vi "Plate Tank 6.vi"() -> ()   [LabVIEW 2019]
uses:
  <vilib>/NI/Current Value Table/Type Defs/Single Tag.ctl
  <vilib>/NI/Current Value Table/Type Defs/Data Types.ctl
  <vilib>/NI/STM/TCP/Read Meta Data (TCP Ref).vi
  <vilib>/NI/STM/TCP/Get Connection Reference (TCP).vi
  <vilib>/NI/AMC/Read Termination Message.vi
  <vilib>/NI/AMC/Create Single Message.vi
  <vilib>/NI/AMC/Update Message Routing Info.vi
  <vilib>/NI/STM/TCP/Read Meta Data (TCP Clst).vi
  <vilib>/NI/AMC/Send Message.vi
  <vilib>/NI/AMC/Globals.vi
  <userlib>/_OpenG.lib/comparison/comparison.llb/I32 Changed__ogtk.vi
  <vilib>/NI/STM/TCP/Write Message (TCP).vi
  <vilib>/NI/AMC/AMC.lvlib
  <vilib>/NI/STM/NI STM.lvlib
  <vilib>/NI/Current Value Table/Current Value Table.lvlib
panel:
  out "Loaded Recipe":string
  in  "Override Motion":bool
  in  "Reverse Current Multiplier":dbl=3.0 min=0.1 max=100.0 step=0.01 format="%.2g"
  in  "Load A Recipe":bool
  in  "Save This Recipe":bool
  out "Right Time":dbl format="%.1f"
  out "Left Time":dbl format="%.1f"
  out "Total Amp*min R":dbl format="%.1f"
  out "Total Amp*min L":dbl format="%.1f"
  in  "Rectifer Settings":i32(listbox)
  in  "MO":string
  in  "BasT1_P Last Hr":bool
  in  "BasT1_Level Last Hr":bool
  out "Boolean 5":bool
  out "SumpBottom":bool
  out "Process 1 Supply":bool
  out "Sump Return":bool
  out "Boolean 2":bool
  out "SG":dbl format="%.3g"
  out "Return to sump 4":bool
  in  "Rectifer Data":enum32{"Standard", "Eng"}(tab)
  out "Current Step":i32
  out "Left Anode Actual Current":dbl(knob) scale=0.0..150.0
  out "Right Anode Actual Current":dbl(knob) scale=0.0..150.0
  out "Left Anode Amp-min":dbl(slide) scale=0.0..800.0
  out "Right Anode Amp-min":dbl(slide) scale=0.0..233.60000610351562
  out "Output Voltage":cluster{dbl, dbl}(graph)
  in  "Tab Control 2":enum32{"Standard", "ENG"}(tab)
  in  "Level Last Hr":bool
  out "Supply Flow":dbl(knob) scale=0.0..65.0
  out "Plating Cell Liquid Level":dbl(slide) scale=0.0..75.0
  out "Cell Temperature":dbl(slide) scale=0.0..60.0
  in  "Cell T Last Hr":bool
  out "Suck Pump":bool
  out "Suck Pump Flow":dbl format="%#_4g"
  out "SuckPipe":bool
  out "SuckPipe 3":bool
  out "Drain Tee Top":bool
  out "Return to sump 2":bool
  out "Return to sump 3":bool
  in  "Supply Tot FlwLast Hr":bool
  in  "Suck FlwLast Hr":bool
  out "Flow Controller":dbl(knob) scale=0.0..100.0
  in  "Tab Control":enum32{"Main Pump", "Suck Pump"}(tab)
  out "Amps":dbl format="%#.2g"
  out "Volts":dbl format="%#.1f"
  out "VFD T":dbl format="%#.2g"
  out "RPM":dbl format="%#.0f"
  out "Fault Code":dbl format="%#.2g"
  out "Freq":dbl format="%#.2g"
  out "SP1 Amps":dbl caption="Amps" format="%#.2g"
  out "SP1 Volts":dbl caption="Volts" format="%#.1g"
  out "SP1 RPM":dbl caption="RPM" format="%#.2g"
  out "SP1 VFD T":dbl caption="VFD T" format="%#.2g"
  out "SP1 Fault Code":dbl caption="Fault Code" format="%#.2g"
  out "SP1 Freq":dbl caption="Freq" format="%#.2g"
  out "Flow 1":dbl format="%#_4g"
  out "Flow 2":dbl format="%#_4g"
  out "Flow 3":dbl format="%#_4g"
  out "Flow 4":dbl format="%#_4g"
  out "Return to sump":bool
  out "E Stop":bool
  out "Run Enabled?":bool
  in  "Full Drain Plating Cell":bool
  out "Rack Motion":bool
  out "Right Eductor Motion":bool
  out "Left Eductor Motion":bool
  out "Right Output On":bool
  in  "Enable Rack Motion":bool
  in  "Rack RPM":dbl(knob) scale=0.0..15.0
  out "Left Output On":bool
  in  "Start Cycle":bool
  in  "Cancel Cycle":bool
  out "SuckPipe 2":bool
  out "Main Pump":bool
  in  "Enable Eductor Motion":bool
  in  "Eductor RPM":dbl(knob) scale=0.0..15.0
  in  "Supply Pressure (kPa)":dbl(knob)=50.0 min=50.0 max=200.0 step=5.0 scale=50.0..200.0
  in  "Total Inflow (L/min)":dbl(knob)=40.0 min=25.0 max=50.0 step=0.5 scale=25.0..50.0
  in  "Suck Pump fraction of inflow":dbl(knob)=5.0 min=5.0 max=90.0 step=1.0 scale=0.0..90.0
  out "Sump Level":dbl(slide) scale=0.0..1000.0
  out "Supply Pressure":dbl(knob) scale=0.0..200.0
  in  "Enable Suck Pump":bool
  in  "Enable Plating Cell":bool
  in  "Machine":bool
  in  "Basement 4":bool
  in  "Dryer":bool
  in  "Rinse 4":bool
  in  "Rinse 3":bool
  in  "Rinse 2":bool
  in  "Basement 3":bool
  in  "Basement 2":bool
  in  "Basement 1":bool
  in  "Plater 6":bool
  in  "Plater 5":bool
  in  "Plater 4":bool
  in  "Plater 3":bool
  in  "Plater 2":bool
  in  "Plater 1":bool
  in  "Predip":bool
  in  "Rinse 1":bool
  in  "Cleaner":bool
  in  "Etch":bool
  out "status":string
  out "Boolean 4":bool
  # "Module Selection"
  # "Rectifier Settings"
  # "Fluid Flow Control"
  # "Rectifier Control"
  # "Rectifier Output"
  # "Note: RPM settings shared with tank 6"
  # "Motion starts when rectifiers cycle"
  # "kPa"
  # "@"
  # "Output"
  # "cm"
  # "°C"
  # "L/min"
  # "cm"
  # "L/min"
  # "L/min"
  # "L/min"
  # "L/min"
  # "L/min"
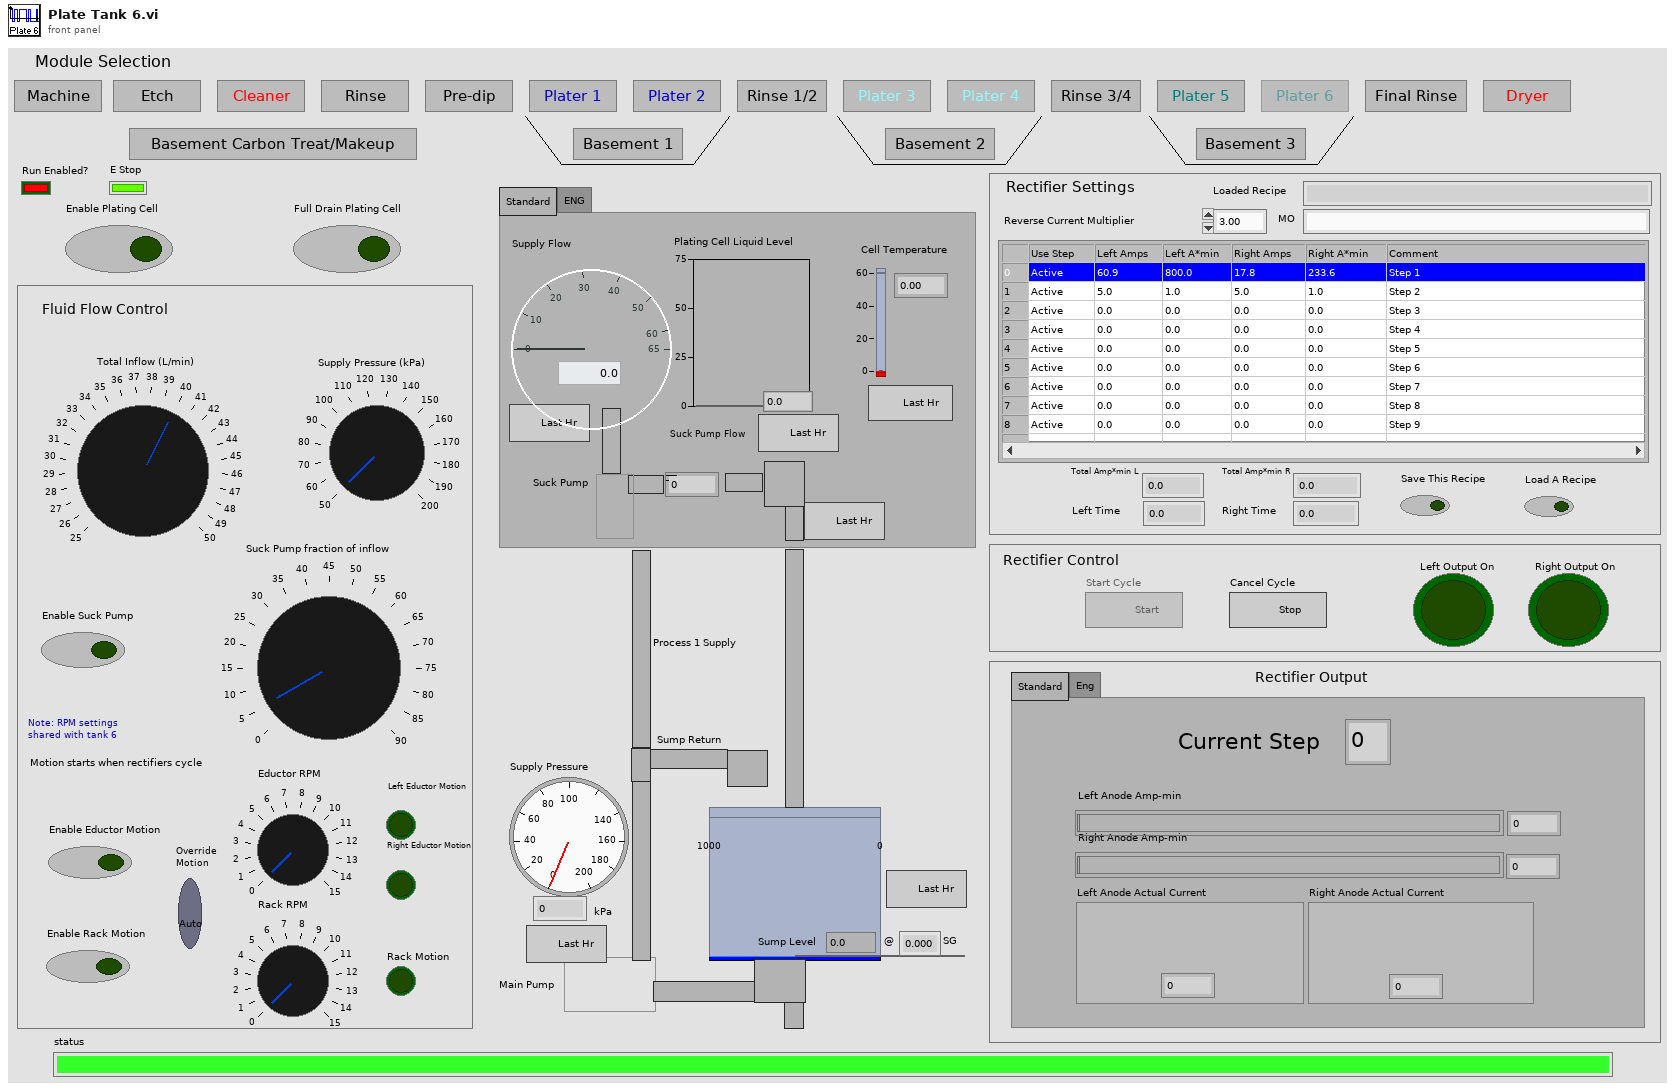
[diagram p1: front panel]
types:
  T1 = typedef "Current Value Table.lvlib/Single Tag.ctl" = cluster{"Data Type":T2, "Name":string, "Value":string, "Description":string}
  T2 = typedef "Current Value Table.lvlib/Data Types.ctl" = enum16{"Double", "Single", "I64", "I32", "I16", "I8", "U64", "U32", "U16", "U8", "String", "Boolean", "Array of U8", "Array of U16", "Array of U32", "Array of U64", "Array of I64", "Array of I32", "Array of I16", "Array of I8", "Array of Double", "Array of Single", "Array of Boolean", "Array of String"}
  T3 = typedef "NI STM.lvlib/TCP Connection Info.ctl" = cluster{"connection ID":refnum<k5>, "meta data":T4[]}
  T4 = typedef "NI STM.lvlib/MetaDataElement.ctl" = string
  T5 = typedef "AMC.lvlib/Message Queue.ctl" = refnum<queue>
  T6 = cluster{"Shift":bool, "Ctrl":bool, "Alt":bool, "Cmd":bool, "Opt":bool}
  T7 = typedef "LVPoint32TypeDef.ctl" = cluster{"Horizontal":i32, "Vertical":i32}
  T8 = typedef "LVRowAndColumnTypeDef.ctl" = cluster{"Row":i32, "Column":i32}
  T9 = enum8{"Enabled", "Disabled", "Disabled and Grayed Out"}
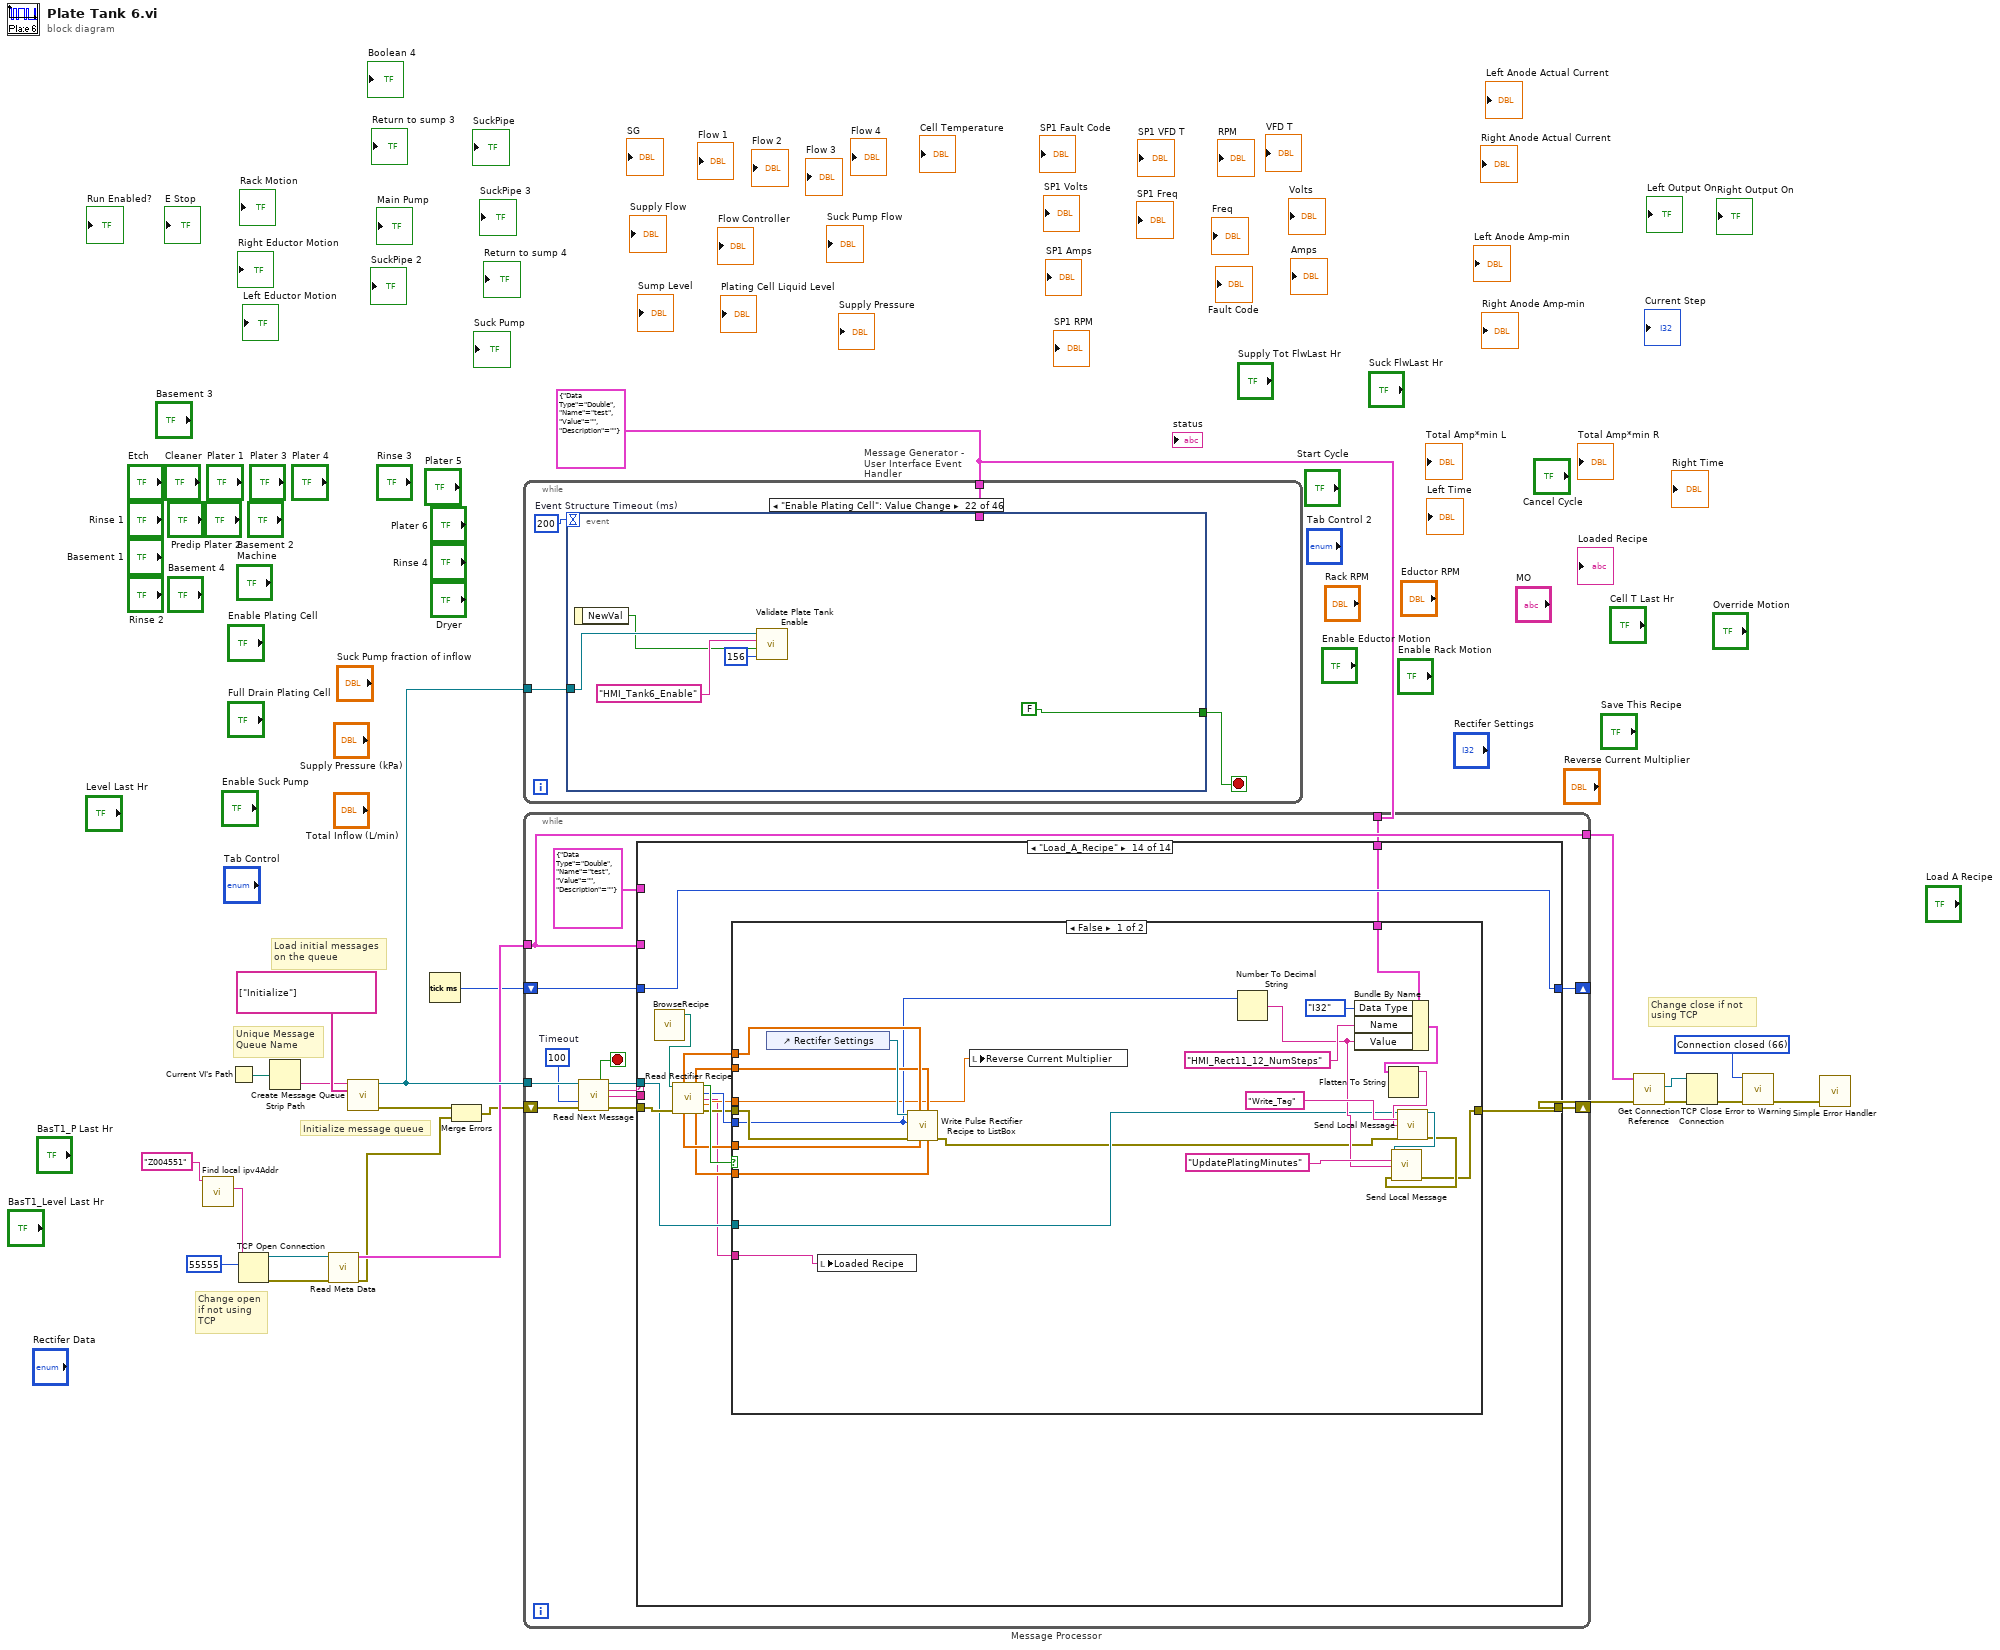
[diagram p0: block diagram]
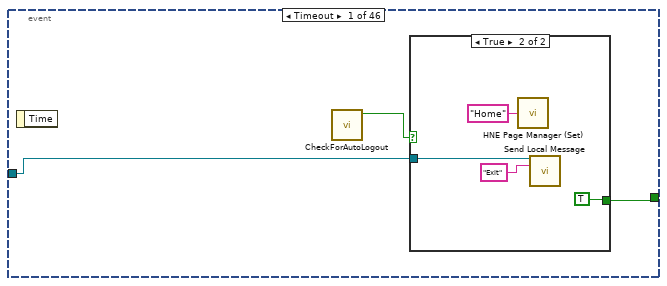
[diagram p2: hidden frame]
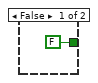
[diagram p3: hidden frame]
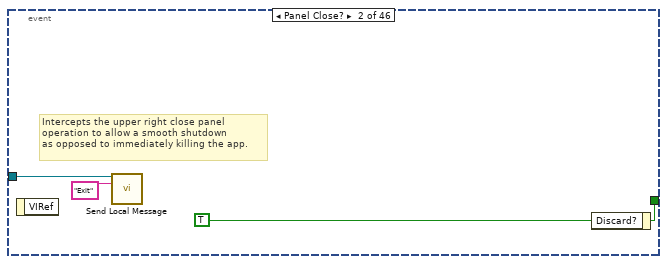
[diagram p4: hidden frame]
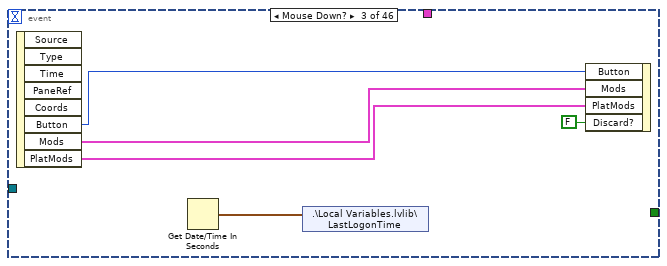
[diagram p5: hidden frame]
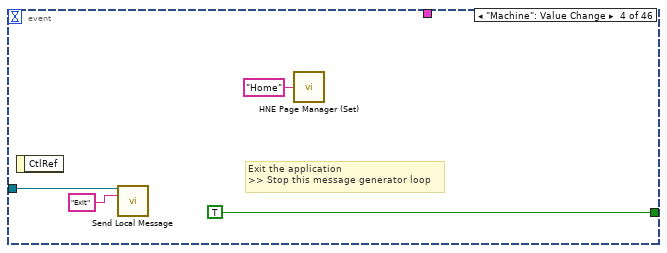
[diagram p6: hidden frame]
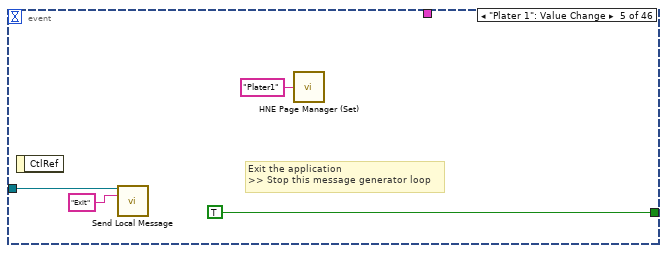
[diagram p7: hidden frame]
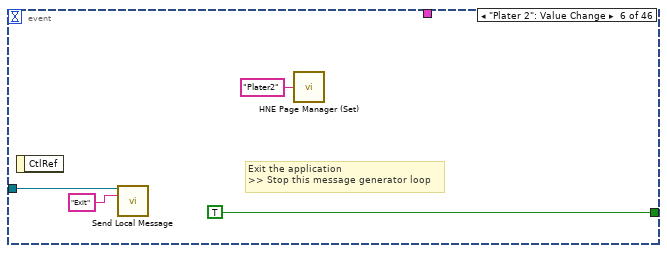
[diagram p8: hidden frame]
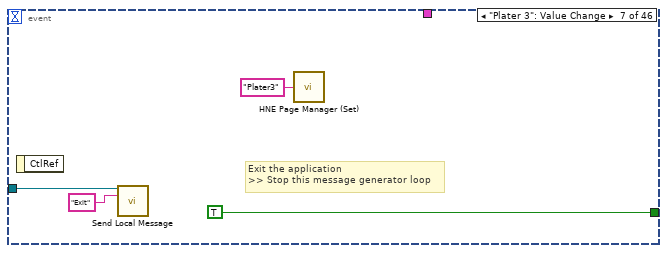
[diagram p9: hidden frame]
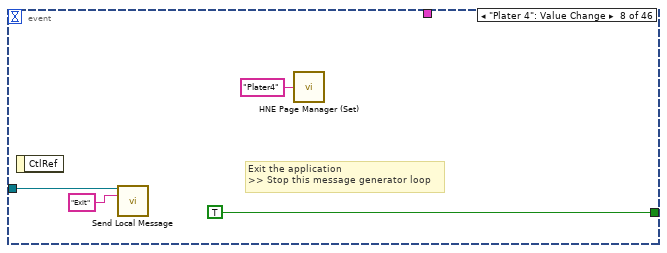
[diagram p10: hidden frame]
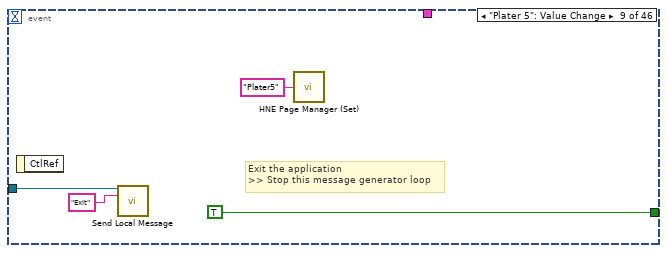
[diagram p11: hidden frame]
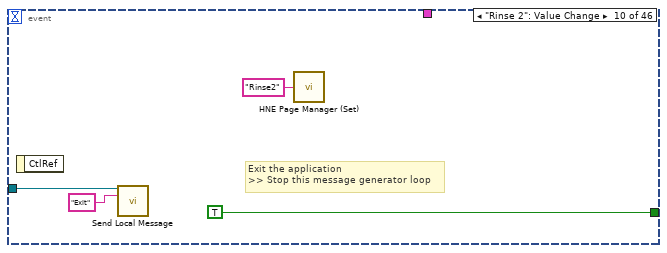
[diagram p12: hidden frame]
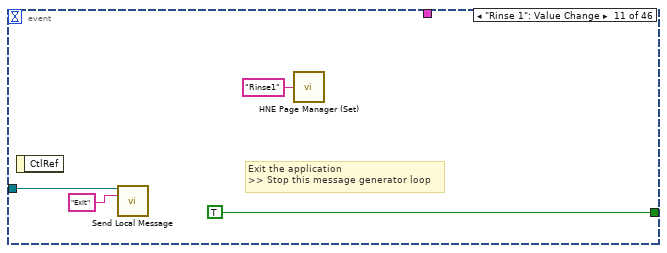
[diagram p13: hidden frame]
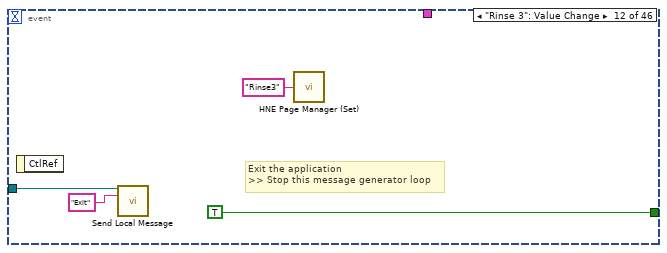
[diagram p14: hidden frame]
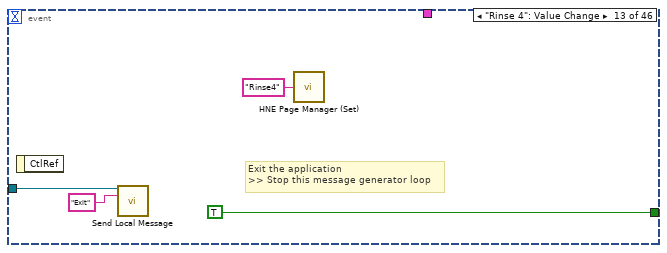
[diagram p15: hidden frame]
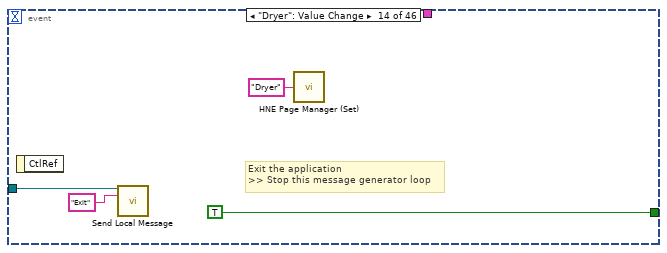
[diagram p16: hidden frame]
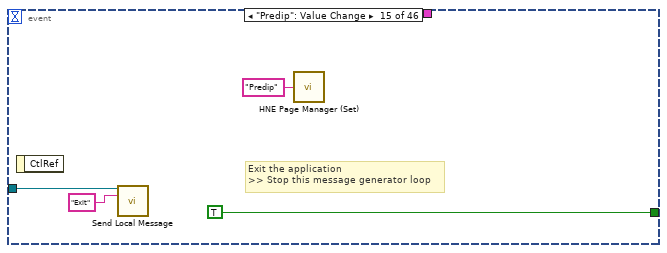
[diagram p17: hidden frame]
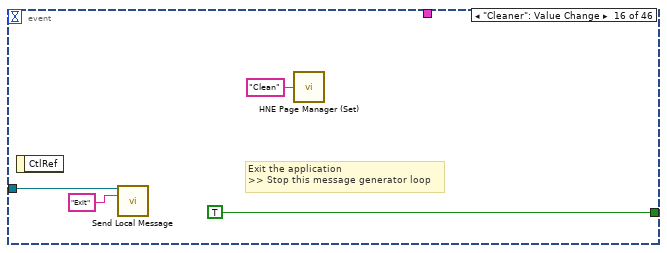
[diagram p18: hidden frame]
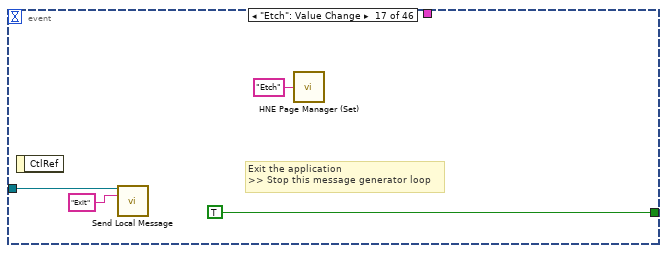
[diagram p19: hidden frame]
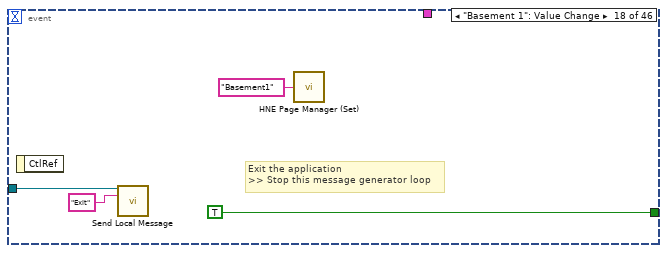
[diagram p20: hidden frame]
diagram:
  w1 = T1 {"Data Type"=enum."Double", "Name"="test", "Value"="", "Description"=""} ("Tag")
  w13 = 66 items=["No Error", "Argument Error", "Memory Full", "Out of Zone", "End of File", "File Already Open", "Generic File IO Error", "File Not Found", "File Permission Error", "Disk Full", "Duplicate Path", "Too Many Files Open", "Not Enabled", "Resource File Not Found", "Cannot Add Resource", "Resource Not Found", "Image Not Found", "Image Memory Error", "Pen Does Not Exist", "Config Bad Type", "Config Token Not Found", "Config Parse Error", "Config Memory Error", "Bad External Code Format", "Bad External Code Offset", "External Code Not Present", "Null Window", "Destroy Window Mixup", "Null Menu", "Print Aborted", "Bad Print Record", "Print Driver Error", "Windows Error During Print", "Memory Error During Print", "Print Dialog Error", "Generic Print Error", "Invalid Device Refnum", "Device Not Found", "Device Parameter Error", "Device Unit Error", "Can't Open Device", "Device Call Aborted", "Generic Error", "Cancelled By User", "Object ID Too Low", "Object ID Too High", "Object Not In Heap", "Unknown Heap", "Bad DefProc ID", "DefProc Not In Table", "Message Out Of Range", "Null Method", "Unknown Message", "Manager Call Not Supported", "Bad address", "Connection In progress", "Connection timed out", "Connection is already in progress", "Network attribute not supported", "Network error", "Address in use", "System out of memory", "Connection aborted", "Connection refused", "Connection is not connected", "Connection is already connected", "Connection closed", "Initialize error (interapplication manager)", "Bad occurrence", "Wait on unbound occurrence handler", "Occurrence queue overflow", "Bad path", "Semaphore not signaled", "Unrecognized type (interapplication manager)"] ("1st Error to Convert")
  # "Change close if not using TCP"
  # "Change open if not using TCP"
  # "Initialize message queue"
  # "Unique Message\nQueue Name"
  # "Load initial messages\non the queue"
  n1 = call "Find local ipv4Addr.vi"("MachineToFind"="Z004551" ("Target IP Address")) -> ("name"=w5:string)  [unwired: 9 in, 1 out]
  n2 = Current VI's Path() -> (path=w19:path)
  n3 = TCP Open Connection(address=w5, remote port or service name=u16 55555 ("remote port")) -> (connection ID=w17:refnum<k5>, error out=w16:errorcluster)  [unwired: 1 in, 2 out]
  n4 = Strip Path(path=w19) -> (name=w21:string)  [unwired: 1 out]
  n5 = call-poly <vilib>:"Read Meta Data.vi"("error in"=w16, "connection ID"=w17) -> ("error out"=w3:errorcluster, "connection info out"=w15:T3)  [unwired: 7 in, 1 out]
  n6 = call <vilib>:"Create Message Queue.vi"("message queue name"=w21, "initial message names"=string[] ["Initialize"]) -> ("message queue out"=w20:T5, "error out"=w4:errorcluster)  [unwired: 12 in]
  n7 = Tick Count (ms)() -> (millisecond timer value=w7:u32)
  n8 = Merge Errors(w4, w3) -> (w2:errorcluster)
  n9 = while "Message Generator - User Interface Event Handler" {
    tunnel: w20 -> [w24]
    tunnel: w1 -> [w23]
    stop <- w25 stop-if-true
    w26 = 200  # Event Structure Timeout (ms)
    n10 = event shown="[21] \"Enable Plating Cell\": Value Change" {
      selector: _ -> [_ _ _ _ _ _ _ _ _ _ _ _ _ _ _ _ _ _ _ _ _ _ _ _ _ _ _ _ _ _ _ _ _ _ _ _ _ _ _ _ _ _ _ _ _ _]
      dyn-events: _ -> [_ _ _ _ _ _ _ _ _ _ _ _ _ _ _ _ _ _ _ _ _ _ _ _ _ _ _ _ _ _ _ _ _ _ _ _ _ _ _ _ _ _ _ _ _ _]
      timeout: w26 -> [_ _ _ _ _ _ _ _ _ _ _ _ _ _ _ _ _ _ _ _ _ _ _ _ _ _ _ _ _ _ _ _ _ _ _ _ _ _ _ _ _ _ _ _ _ _]
      tunnel: [w29 w37 _ TRUE ("Discard?") TRUE ("Discard?") TRUE ("Discard?") TRUE ("Discard?") TRUE ("Discard?") TRUE ("Discard?") TRUE ("Discard?") TRUE ("Discard?") TRUE ("Discard?") TRUE ("Discard?") TRUE ("Discard?") TRUE ("Discard?") TRUE ("Discard?") TRUE ("Discard?") TRUE ("Discard?") TRUE ("Discard?") TRUE ("Discard?") TRUE ("Discard?") FALSE ("Discard?") FALSE ("Discard?") FALSE ("Discard?") FALSE ("Discard?") FALSE ("Discard?") FALSE ("Discard?") FALSE ("Discard?") FALSE ("Discard?") FALSE ("Discard?") FALSE ("Discard?") FALSE ("Discard?") FALSE ("Discard?") FALSE ("Discard?") FALSE ("Discard?") FALSE ("Discard?") _ _ _ _ _ _ _ _ _ _] -> w25
      tunnel: w24 -> [w28 w35 _ w44 w48 w52 w56 w60 w64 w68 w72 w76 w80 w84 w88 w92 w96 w100 w104 w108 w112 w118 w121 w126 w139 w150 w161 w172 w183 w187 w201 w221 w231 w241 w251 w263 w265 w267 w272 w277 w282 w287 w292 w299 w317 _]
      tunnel: w23 -> [_ _ _ _ _ _ _ _ _ _ _ _ _ _ _ _ _ _ _ _ _ _ _ _ w136 w147 w158 w169 w180 w186 w200 w220 w230 w240 w250 w262 _ _ _ _ _ _ _ w298 _ _]
      event Timeout {
        n11 = event-data() -> ()  [unwired: 2 out]
        n12 = call "CheckForAutoLogout.vi"() -> ("Boolean"=w27:bool)  [unwired: 11 in]
        n13 = case shown="True" w27 {
          tunnel: [FALSE ("Discard?") TRUE ("Discard?")] -> w29
          tunnel: w28 -> [_ w31]
          frame False {
          }
          frame True {
            n14 = call <userlib>:"HNE Page Manager (Set).vi"("Next Page"="Home") -> ()  [unwired: 4 in, 1 out]
            n15 = call <vilib>:"Send Local Message.vi"("message queue in"=w31, "message name"="Exit") -> ()  [unwired: 11 in, 3 out]
          }
        }
      }
      event Panel Close? {
        w37 = TRUE ("Discard?")
        # "Intercepts the upper right close panel\noperation to allow a smooth shutdown\nas opposed to immediately killing the app."
        n16 = event-data() -> ()  [unwired: 2 out]
        n17 = call <vilib>:"Send Local Message.vi"("message queue in"=w35, "message name"="Exit") -> ()  [unwired: 11 in, 3 out]
        n18 = event-data("Discard?"=w37) -> ()  [unwired: 1 in, 1 out]
      }
      event Mouse Down? {
        n19 = event-data() -> ("Button"=w41:u16, "Mods"=w40:cluster{"Double Click":bool, "Menu Key":bool}, "PlatMods"=w39:T6)  [unwired: 6 out]
        n20 = Get Date/Time In Seconds() -> (seconds since 1Jan1904=w38:timestamp)
        n21 = shared-variable ".\\Local Variables.lvlib\\LastLogonTime"(w38) -> ()  [unwired: 1 in, 1 out]
        n22 = event-data("Button"=w41, "Mods"=w40, "PlatMods"=w39, "Discard?"=FALSE) -> ()  [unwired: 1 in, 1 out]
      }
      event "Machine": Value Change {
        # "Exit the application\n>> Stop this message generator loop"
        n23 = event-data() -> ()  [unwired: 2 out]
        n24 = call <vilib>:"Send Local Message.vi"("message queue in"=w44, "message name"="Exit") -> ()  [unwired: 11 in, 3 out]
        n25 = call <userlib>:"HNE Page Manager (Set).vi"("Next Page"="Home") -> ()  [unwired: 4 in, 1 out]
      }
      event "Plater 1": Value Change {
        # "Exit the application\n>> Stop this message generator loop"
        n26 = event-data() -> ()  [unwired: 2 out]
        n27 = call <vilib>:"Send Local Message.vi"("message queue in"=w48, "message name"="Exit") -> ()  [unwired: 11 in, 3 out]
        n28 = call <userlib>:"HNE Page Manager (Set).vi"("Next Page"="Plater1") -> ()  [unwired: 4 in, 1 out]
      }
      event "Plater 2": Value Change {
        # "Exit the application\n>> Stop this message generator loop"
        n29 = event-data() -> ()  [unwired: 2 out]
        n30 = call <vilib>:"Send Local Message.vi"("message queue in"=w52, "message name"="Exit") -> ()  [unwired: 11 in, 3 out]
        n31 = call <userlib>:"HNE Page Manager (Set).vi"("Next Page"="Plater2") -> ()  [unwired: 4 in, 1 out]
      }
      event "Plater 3": Value Change {
        # "Exit the application\n>> Stop this message generator loop"
        n32 = event-data() -> ()  [unwired: 2 out]
        n33 = call <vilib>:"Send Local Message.vi"("message queue in"=w56, "message name"="Exit") -> ()  [unwired: 11 in, 3 out]
        n34 = call <userlib>:"HNE Page Manager (Set).vi"("Next Page"="Plater3") -> ()  [unwired: 4 in, 1 out]
      }
      event "Plater 4": Value Change {
        # "Exit the application\n>> Stop this message generator loop"
        n35 = event-data() -> ()  [unwired: 2 out]
        n36 = call <vilib>:"Send Local Message.vi"("message queue in"=w60, "message name"="Exit") -> ()  [unwired: 11 in, 3 out]
        n37 = call <userlib>:"HNE Page Manager (Set).vi"("Next Page"="Plater4") -> ()  [unwired: 4 in, 1 out]
      }
      event "Plater 5": Value Change {
        # "Exit the application\n>> Stop this message generator loop"
        n38 = event-data() -> ()  [unwired: 2 out]
        n39 = call <vilib>:"Send Local Message.vi"("message queue in"=w64, "message name"="Exit") -> ()  [unwired: 11 in, 3 out]
        n40 = call <userlib>:"HNE Page Manager (Set).vi"("Next Page"="Plater5") -> ()  [unwired: 4 in, 1 out]
      }
      event "Rinse 2": Value Change {
        # "Exit the application\n>> Stop this message generator loop"
        n41 = event-data() -> ()  [unwired: 2 out]
        n42 = call <vilib>:"Send Local Message.vi"("message queue in"=w68, "message name"="Exit") -> ()  [unwired: 11 in, 3 out]
        n43 = call <userlib>:"HNE Page Manager (Set).vi"("Next Page"="Rinse2") -> ()  [unwired: 4 in, 1 out]
      }
      event "Rinse 1": Value Change {
        # "Exit the application\n>> Stop this message generator loop"
        n44 = event-data() -> ()  [unwired: 2 out]
        n45 = call <vilib>:"Send Local Message.vi"("message queue in"=w72, "message name"="Exit") -> ()  [unwired: 11 in, 3 out]
        n46 = call <userlib>:"HNE Page Manager (Set).vi"("Next Page"="Rinse1") -> ()  [unwired: 4 in, 1 out]
      }
      event "Rinse 3": Value Change {
        # "Exit the application\n>> Stop this message generator loop"
        n47 = event-data() -> ()  [unwired: 2 out]
        n48 = call <vilib>:"Send Local Message.vi"("message queue in"=w76, "message name"="Exit") -> ()  [unwired: 11 in, 3 out]
        n49 = call <userlib>:"HNE Page Manager (Set).vi"("Next Page"="Rinse3") -> ()  [unwired: 4 in, 1 out]
      }
      event "Rinse 4": Value Change {
        # "Exit the application\n>> Stop this message generator loop"
        n50 = event-data() -> ()  [unwired: 2 out]
        n51 = call <vilib>:"Send Local Message.vi"("message queue in"=w80, "message name"="Exit") -> ()  [unwired: 11 in, 3 out]
        n52 = call <userlib>:"HNE Page Manager (Set).vi"("Next Page"="Rinse4") -> ()  [unwired: 4 in, 1 out]
      }
      event "Dryer": Value Change {
        # "Exit the application\n>> Stop this message generator loop"
        n53 = event-data() -> ()  [unwired: 2 out]
        n54 = call <vilib>:"Send Local Message.vi"("message queue in"=w84, "message name"="Exit") -> ()  [unwired: 11 in, 3 out]
        n55 = call <userlib>:"HNE Page Manager (Set).vi"("Next Page"="Dryer") -> ()  [unwired: 4 in, 1 out]
      }
      event "Predip": Value Change {
        # "Exit the application\n>> Stop this message generator loop"
        n56 = event-data() -> ()  [unwired: 2 out]
        n57 = call <vilib>:"Send Local Message.vi"("message queue in"=w88, "message name"="Exit") -> ()  [unwired: 11 in, 3 out]
        n58 = call <userlib>:"HNE Page Manager (Set).vi"("Next Page"="Predip") -> ()  [unwired: 4 in, 1 out]
      }
      event "Cleaner": Value Change {
        # "Exit the application\n>> Stop this message generator loop"
        n59 = event-data() -> ()  [unwired: 2 out]
        n60 = call <vilib>:"Send Local Message.vi"("message queue in"=w92, "message name"="Exit") -> ()  [unwired: 11 in, 3 out]
        n61 = call <userlib>:"HNE Page Manager (Set).vi"("Next Page"="Clean") -> ()  [unwired: 4 in, 1 out]
      }
      event "Etch": Value Change {
        # "Exit the application\n>> Stop this message generator loop"
        n62 = event-data() -> ()  [unwired: 2 out]
        n63 = call <vilib>:"Send Local Message.vi"("message queue in"=w96, "message name"="Exit") -> ()  [unwired: 11 in, 3 out]
        n64 = call <userlib>:"HNE Page Manager (Set).vi"("Next Page"="Etch") -> ()  [unwired: 4 in, 1 out]
      }
      event "Basement 1": Value Change {
        # "Exit the application\n>> Stop this message generator loop"
        n65 = event-data() -> ()  [unwired: 2 out]
        n66 = call <vilib>:"Send Local Message.vi"("message queue in"=w100, "message name"="Exit") -> ()  [unwired: 11 in, 3 out]
        n67 = call <userlib>:"HNE Page Manager (Set).vi"("Next Page"="Basement1") -> ()  [unwired: 4 in, 1 out]
      }
      event "Basement 2": Value Change {
        # "Exit the application\n>> Stop this message generator loop"
        n68 = event-data() -> ()  [unwired: 2 out]
        n69 = call <vilib>:"Send Local Message.vi"("message queue in"=w104, "message name"="Exit") -> ()  [unwired: 11 in, 3 out]
        n70 = call <userlib>:"HNE Page Manager (Set).vi"("Next Page"="Basement2") -> ()  [unwired: 4 in, 1 out]
      }
      event "Basement 3": Value Change {
        # "Exit the application\n>> Stop this message generator loop"
        n71 = event-data() -> ()  [unwired: 2 out]
        n72 = call <vilib>:"Send Local Message.vi"("message queue in"=w108, "message name"="Exit") -> ()  [unwired: 11 in, 3 out]
        n73 = call <userlib>:"HNE Page Manager (Set).vi"("Next Page"="Basement3") -> ()  [unwired: 4 in, 1 out]
      }
      event "Basement 4": Value Change {
        # "Exit the application\n>> Stop this message generator loop"
        n74 = event-data() -> ()  [unwired: 2 out]
        n75 = call <vilib>:"Send Local Message.vi"("message queue in"=w112, "message name"="Exit") -> ()  [unwired: 11 in, 3 out]
        n76 = call <userlib>:"HNE Page Manager (Set).vi"("Next Page"="Basement4") -> ()  [unwired: 4 in, 1 out]
      }
      event "Enable Plating Cell": Value Change {
        n77 = event-data() -> ("NewVal"=w116:bool)  [unwired: 1 out]
        n78 = call "Validate Plate Tank Enable.vi"("Valve No."=156, "Test Value"=w116, "Tag"="HMI_Tank6_Enable", "Queue in"=w118) -> ()  [unwired: 8 in]
      }
      event "Save This Recipe": Value Change {
        n79 = event-data() -> ("NewVal"=w120:bool)  [unwired: 1 out]
        n80 = case shown="True" w120 {
          tunnel: w121 -> [_ w123]
          frame False {
          }
          frame True {
            n81 = call <vilib>:"Send Local Message.vi"("message queue in"=w123, "message name"="Save_Recipe") -> ()  [unwired: 11 in, 3 out]
          }
        }
      }
      event "Load A Recipe": Value Change {
        n82 = event-data() -> ("NewVal"=w125:bool)  [unwired: 1 out]
        n83 = case shown="True" w125 {
          tunnel: w126 -> [_ w128]
          frame False {
          }
          frame True {
            n84 = call <vilib>:"Send Local Message.vi"("message queue in"=w128, "message name"="Load_A_Recipe") -> ()  [unwired: 11 in, 3 out]
          }
        }
      }
      event "Full Drain Plating Cell": Value Change {
        n85 = event-data() -> ("NewVal"=w138:bool)  [unwired: 1 out]
        n86 = Boolean To (0,1)(Boolean=w138) -> (0, 1=w137:i16)
        n87 = Number To Decimal String(number=w137) -> (decimal integer string=w133:string)  [unwired: 1 in]
        n88 = Bundle By Name(cluster=w136, "Data Type"=Data_Types."Boolean", "Name"="HMI_Tank6_Drain", "Value"=w133) -> (w132:T1)
        n89 = Flatten To String(anything=w132) -> (data string=w131:string)  [unwired: 3 in, 2 out]
        n90 = call <vilib>:"Send Local Message.vi"("message queue in"=w139, "message name"="Write_Tag", "message value"=w131) -> ()  [unwired: 10 in, 3 out]
      }
      event "Enable Eductor Motion": Value Change {
        n91 = event-data() -> ("NewVal"=w149:bool)  [unwired: 1 out]
        n92 = Boolean To (0,1)(Boolean=w149) -> (0, 1=w148:i16)
        n93 = Number To Decimal String(number=w148) -> (decimal integer string=w144:string)  [unwired: 1 in]
        n94 = Bundle By Name(cluster=w147, "Data Type"=Data_Types."Boolean", "Name"="HMI_Tank6_Eductor_Motors_Run", "Value"=w144) -> (w143:T1)
        n95 = Flatten To String(anything=w143) -> (data string=w142:string)  [unwired: 3 in, 2 out]
        n96 = call <vilib>:"Send Local Message.vi"("message queue in"=w150, "message name"="Write_Tag", "message value"=w142) -> ()  [unwired: 10 in, 3 out]
      }
      event "Enable Rack Motion": Value Change {
        n97 = event-data() -> ("NewVal"=w160:bool)  [unwired: 1 out]
        n98 = Boolean To (0,1)(Boolean=w160) -> (0, 1=w159:i16)
        n99 = Number To Decimal String(number=w159) -> (decimal integer string=w155:string)  [unwired: 1 in]
        n100 = Bundle By Name(cluster=w158, "Data Type"=Data_Types."Boolean", "Name"="HMI_Tank6_Rack_Motor_Run", "Value"=w155) -> (w154:T1)
        n101 = Flatten To String(anything=w154) -> (data string=w153:string)  [unwired: 3 in, 2 out]
        n102 = call <vilib>:"Send Local Message.vi"("message queue in"=w161, "message name"="Write_Tag", "message value"=w153) -> ()  [unwired: 10 in, 3 out]
      }
      event "Enable Suck Pump": Value Change {
        n103 = event-data() -> ("NewVal"=w171:bool)  [unwired: 1 out]
        n104 = Boolean To (0,1)(Boolean=w171) -> (0, 1=w170:i16)
        n105 = Number To Decimal String(number=w170) -> (decimal integer string=w166:string)  [unwired: 1 in]
        n106 = Bundle By Name(cluster=w169, "Data Type"=Data_Types."Boolean", "Name"="HMI_Tnk6_Enable_SuckPump", "Value"=w166) -> (w165:T1)
        n107 = Flatten To String(anything=w165) -> (data string=w164:string)  [unwired: 3 in, 2 out]
        n108 = call <vilib>:"Send Local Message.vi"("message queue in"=w172, "message name"="Write_Tag", "message value"=w164) -> ()  [unwired: 10 in, 3 out]
      }
      event "Override Motion": Value Change {
        n109 = event-data() -> ("NewVal"=w182:bool)  [unwired: 1 out]
        n110 = Boolean To (0,1)(Boolean=w182) -> (0, 1=w181:i16)
        n111 = Number To Decimal String(number=w181) -> (decimal integer string=w177:string)  [unwired: 1 in]
        n112 = Bundle By Name(cluster=w180, "Data Type"=Data_Types."Boolean", "Name"="HMI_Tank6_Motion_OverRide", "Value"=w177) -> (w176:T1)
        n113 = Flatten To String(anything=w176) -> (data string=w175:string)  [unwired: 3 in, 2 out]
        n114 = call <vilib>:"Send Local Message.vi"("message queue in"=w183, "message name"="Write_Tag", "message value"=w175) -> ()  [unwired: 10 in, 3 out]
      }
      event "Start Cycle": Value Change {
        n115 = event-data() -> ("NewVal"=w185:bool)  [unwired: 1 out]
        n116 = case shown="True" w185 {
          tunnel: w187 -> [_ w198]
          tunnel: w185 -> [_ w197]
          tunnel: w186 -> [_ w195]
          frame False {
          }
          frame True {
            n117 = Boolean To (0,1)(Boolean=w197) -> (0, 1=w196:i16)
            n118 = Number To Decimal String(number=w196) -> (decimal integer string=w192:string)  [unwired: 1 in]
            n119 = Bundle By Name(cluster=w195, "Data Type"=Data_Types."Boolean", "Name"="HMI_Rect11_12_Cycle", "Value"=w192) -> (w191:T1)
            n120 = Flatten To String(anything=w191) -> (data string=w190:string)  [unwired: 3 in, 2 out]
            n121 = call <vilib>:"Send Local Message.vi"("message queue in"=w198, "message name"="Write_Tag", "message value"=w190) -> ()  [unwired: 10 in, 3 out]
          }
        }
      }
      event "Cancel Cycle": Value Change {
        n122 = event-data() -> ("NewVal"=w199:bool)  [unwired: 1 out]
        n123 = case shown="True" w199 {
          tunnel: w201 -> [_ w212]
          tunnel: w199 -> [_ w211]
          tunnel: w200 -> [_ w209]
          frame False {
          }
          frame True {
            n124 = Boolean To (0,1)(Boolean=w211) -> (0, 1=w210:i16)
            n125 = Number To Decimal String(number=w210) -> (decimal integer string=w206:string)  [unwired: 1 in]
            n126 = Bundle By Name(cluster=w209, "Data Type"=Data_Types."Boolean", "Name"="HMI_Rect11_12_CycleStop", "Value"=w206) -> (w205:T1)
            n127 = Flatten To String(anything=w205) -> (data string=w204:string)  [unwired: 3 in, 2 out]
            n128 = call <vilib>:"Send Local Message.vi"("message queue in"=w212, "message name"="Write_Tag", "message value"=w204) -> ()  [unwired: 10 in, 3 out]
          }
        }
      }
      event "Eductor RPM": Value Change {
        n129 = event-data() -> ("NewVal"=w214:dbl)  [unwired: 1 out]
        n130 = Number To Fractional String(number=w214) -> (F-format string=w213:string)  [unwired: 3 in]
        n131 = Bundle By Name(cluster=w220, "Data Type"=Data_Types."Double", "Name"="HMI_Tnk5_Eductor_RPM", "Value"=w213) -> (w217:T1)
        n132 = Flatten To String(anything=w217) -> (data string=w216:string)  [unwired: 3 in, 2 out]
        n133 = call <vilib>:"Send Local Message.vi"("message queue in"=w221, "message name"="Write_Tag", "message value"=w216) -> ()  [unwired: 10 in, 3 out]
      }
      event "Rack RPM": Value Change {
        n134 = event-data() -> ("NewVal"=w224:dbl)  [unwired: 1 out]
        n135 = Number To Fractional String(number=w224) -> (F-format string=w223:string)  [unwired: 3 in]
        n136 = Bundle By Name(cluster=w230, "Data Type"=Data_Types."Double", "Name"="HMI_Tnk5_Rack_RPM", "Value"=w223) -> (w227:T1)
        n137 = Flatten To String(anything=w227) -> (data string=w226:string)  [unwired: 3 in, 2 out]
        n138 = call <vilib>:"Send Local Message.vi"("message queue in"=w231, "message name"="Write_Tag", "message value"=w226) -> ()  [unwired: 10 in, 3 out]
      }
      event "Total Inflow (L/min)": Value Change {
        n139 = event-data() -> ("NewVal"=w234:dbl)  [unwired: 1 out]
        n140 = Number To Fractional String(number=w234) -> (F-format string=w233:string)  [unwired: 3 in]
        n141 = Bundle By Name(cluster=w240, "Data Type"=Data_Types."Double", "Name"="HMI_TNK6_Flow_Setpoint", "Value"=w233) -> (w237:T1)
        n142 = Flatten To String(anything=w237) -> (data string=w236:string)  [unwired: 3 in, 2 out]
        n143 = call <vilib>:"Send Local Message.vi"("message queue in"=w241, "message name"="Write_Tag", "message value"=w236) -> ()  [unwired: 10 in, 3 out]
      }
      event "Supply Pressure (kPa)": Value Change {
        n144 = event-data() -> ("NewVal"=w244:dbl)  [unwired: 1 out]
        n145 = Number To Fractional String(number=w244) -> (F-format string=w243:string)  [unwired: 3 in]
        n146 = Bundle By Name(cluster=w250, "Data Type"=Data_Types."Double", "Name"="HMI_BAS_TNK3_P_Setpoint", "Value"=w243) -> (w247:T1)
        n147 = Flatten To String(anything=w247) -> (data string=w246:string)  [unwired: 3 in, 2 out]
        n148 = call <vilib>:"Send Local Message.vi"("message queue in"=w251, "message name"="Write_Tag", "message value"=w246) -> ()  [unwired: 10 in, 3 out]
      }
      event "Suck Pump fraction of inflow": Value Change {
        n149 = event-data() -> ("NewVal"=w254:dbl)  [unwired: 1 out]
        n150 = Divide(x=w254, y=100.0) -> (x/y=w253:dbl)
        n151 = Number To Fractional String(number=w253) -> (F-format string=w256:string)  [unwired: 3 in]
        n152 = Bundle By Name(cluster=w262, "Data Type"=Data_Types."Double", "Name"="HMI_TNK6_SuckPmpFrac_Setpoint", "Value"=w256) -> (w259:T1)
        n153 = Flatten To String(anything=w259) -> (data string=w258:string)  [unwired: 3 in, 2 out]
        n154 = call <vilib>:"Send Local Message.vi"("message queue in"=w263, "message name"="Write_Tag", "message value"=w258) -> ()  [unwired: 10 in, 3 out]
      }
      event Menu Selection (User) {
        # "Add run-time menu items to the message\nqueue. The message handler case names must match the menu ItemTag names."
        n155 = event-data() -> ("ItemTag"=w266:string)  [unwired: 1 out]
        n156 = call <vilib>:"Send Local Message.vi"("message queue in"=w265, "message name"=w266) -> ()  [unwired: 11 in, 3 out]
      }
      event "Cell T Last Hr": Value Change {
        n157 = event-data() -> ("NewVal"=w268:bool)  [unwired: 3 out]
        n158 = case shown="True" w268 {
          tunnel: w267 -> [_ w271]
          frame False {
          }
          frame True {
            n159 = call <vilib>:"Send Local Message.vi"("message queue in"=w271, "message name"="DisplayLastHr", "message value"="TNK6_Temperature") -> ()  [unwired: 10 in, 3 out]
          }
        }
      }
      event "BasT1_Level Last Hr": Value Change {
        n160 = event-data() -> ("NewVal"=w273:bool)  [unwired: 3 out]
        n161 = case shown="True" w273 {
          tunnel: w272 -> [_ w276]
          frame False {
          }
          frame True {
            n162 = call <vilib>:"Send Local Message.vi"("message queue in"=w276, "message name"="DisplayLastHr", "message value"="BAS_Proc3_Tank_Level") -> ()  [unwired: 10 in, 3 out]
          }
        }
      }
      event "BasT1_P Last Hr": Value Change {
        n163 = event-data() -> ("NewVal"=w278:bool)  [unwired: 3 out]
        n164 = case shown="True" w278 {
          tunnel: w277 -> [_ w281]
          frame False {
          }
          frame True {
            n165 = call <vilib>:"Send Local Message.vi"("message queue in"=w281, "message name"="DisplayLastHr", "message value"="TNK56_MainPressure") -> ()  [unwired: 10 in, 3 out]
          }
        }
      }
      event "Supply Tot FlwLast Hr": Value Change {
        n166 = event-data() -> ("NewVal"=w283:bool)  [unwired: 3 out]
        n167 = case shown="True" w283 {
          tunnel: w282 -> [_ w286]
          frame False {
          }
          frame True {
            n168 = call <vilib>:"Send Local Message.vi"("message queue in"=w286, "message name"="DisplayLastHr", "message value"="Proc6_Total_Flow") -> ()  [unwired: 10 in, 3 out]
          }
        }
      }
      event "Suck FlwLast Hr": Value Change {
        n169 = event-data() -> ("NewVal"=w288:bool)  [unwired: 3 out]
        n170 = case shown="True" w288 {
          tunnel: w287 -> [_ w291]
          frame False {
          }
          frame True {
            n171 = call <vilib>:"Send Local Message.vi"("message queue in"=w291, "message name"="DisplayLastHr", "message value"="TNK6_SuckFlow") -> ()  [unwired: 10 in, 3 out]
          }
        }
      }
      event "Level Last Hr": Value Change {
        n172 = event-data() -> ("NewVal"=w293:bool)  [unwired: 3 out]
        n173 = case shown="True" w293 {
          tunnel: w292 -> [_ w296]
          frame False {
          }
          frame True {
            n174 = call <vilib>:"Send Local Message.vi"("message queue in"=w296, "message name"="DisplayLastHr", "message value"="TNK6_Level") -> ()  [unwired: 10 in, 3 out]
          }
        }
      }
      event "Rectifer Settings": Mouse Down {
        n175 = event-data() -> ("CtlRef"=w303:refnum<vi>, "Coords"=w301:T7, "Button"=w302:u16)  [unwired: 6 out]
        n176 = call "Handle Rectifer Step Selection.vi"("Coords"=w301, "Button"=w302, "MulticolumnListbox in"=w303) -> ("Row"=w297:i32)  [unwired: 8 in]
        n177 = Greater Than 0?(x=w297) -> (x > 0?=w300:bool)
        n178 = case shown="True" w300 {
          tunnel: w299 -> [_ w306]
          tunnel: w298 -> [_ w305]
          tunnel: w297 -> [_ w304]
          frame False {
          }
          frame True {
            n179 = Number To Decimal String(number=w304) -> (decimal integer string=w307:string)  [unwired: 1 in]
            n180 = Bundle By Name(cluster=w305, "Data Type"=Data_Types."I32", "Name"="HMI_Rect11_12_NumSteps", "Value"=w307) -> (w311:T1)
            n181 = Flatten To String(anything=w311) -> (data string=w310:string)  [unwired: 3 in, 2 out]
            n182 = call <vilib>:"Send Local Message.vi"("message queue in"=w306, "message name"="Write_Tag", "message value"=w310) -> ("message queue out"=w309:T5)  [unwired: 10 in, 2 out]
            n183 = call <vilib>:"Send Local Message.vi"("message queue in"=w309, "message name"="UpdatePlatingMinutes", "message value"=w307) -> ()  [unwired: 10 in, 3 out]
          }
        }
      }
      event "Rectifer Settings": Edit Cell {
        n184 = event-data() -> ("CtlRef"=w321:refnum<vi>, "String"=w320:string, "Coords"=w319:T8)  [unwired: 4 out]
        n185 = call "Data Check Rectifier Settings.vi"("String"=w320, "Coords"=w319, "MulticolumnListbox in"=w321) -> ("error out"=w316:errorcluster)  [unwired: 7 in, 1 out]
        n186 = shared-variable-read(refnum<k21> "ni.var.psp://z004551/CDL0100 ReadWriteTags/HMI_Rect11_12_NumSteps" ("shared variable refnum in"), 0) -> (w322:i32)  [unwired: 1 in, 3 out]
        n187 = Number To Decimal String(number=w322) -> (decimal integer string=w315:string)  [unwired: 1 in]
        n188 = call <vilib>:"Send Local Message.vi"("message queue in"=w317, "message name"="UpdatePlatingMinutes", "message value"=w315, "error in"=w316) -> ()  [unwired: 9 in, 3 out]
      }
      event "MO": Value Change {
        n189 = event-data() -> ("NewVal"=w325:string)  [unwired: 6 out]
        n190 = shared-variable ".\\Local Variables.lvlib\\PT6_MO"(w325) -> ()  [unwired: 1 in, 1 out]
      }
    }
  }
  n191 = while "Message Processor" {
    shift-left: w2 -> [w335]
    shift-right: [w339] -> w8
    tunnel: w20 -> [w336]
    tunnel: w15 -> [w330]
    tunnel: [w330] -> w9
    shift-right: [w327] -> _
    shift-left: w7 -> [w328]
    tunnel: w1 -> [w326]
    stop <- w338 stop-if-true
    w331 = 100  # Timeout
    n192 = call <vilib>:"Read Next Message.vi"("message queue in"=w336, "timeout (1 ms)"=w331, "error in"=w335) -> ("exit process?"=w338:bool, "message queue out"=w337:T5, "message name"=w333:string, "message value"=w332:string, "error out"=w334:errorcluster)  [unwired: 5 in, 3 out]
    n193 = case shown="\"Load_A_Recipe\"" w333 {
      selector: w333 -> [_ _ w431 _ _ _ _ _ _ _ _ _ _ _]
      tunnel: w337 -> [_ _ _ _ _ _ w583 _ _ _ _ w605 _ w629]
      tunnel: w334 -> [w340 w352 w432 w433 w435 w437 w584 w586 w590 w593 w595 w609 w623 w640]
      tunnel: [w340 w352 w432 errorcluster {"status"=FALSE, "code"=0, "source"=""} ("error out") w435 w437 w582 w586 w589 w593 w595 w608 w614 w632] -> w339
      tunnel: w332 -> [_ _ _ _ _ _ _ _ w588 _ w597 w600 _ _]
      tunnel: w330 -> [_ _ _ _ _ _ _ _ w591 _ _ _ _ _]
      tunnel: T1 {"Data Type"=enum."Double", "Name"="test", "Value"="", "Description"=""} ("Tag") -> [_ _ _ _ _ _ _ _ _ _ _ _ _ _]
      tunnel: w328 -> [_ w347 _ _ _ w436 _ _ w587 w594 w596 _ w613 w631]
      tunnel: [_ w348 _ _ _ w436 _ _ w587 w594 w596 _ w613 w631] -> w327
      tunnel: w326 -> [_ _ _ _ _ _ _ _ _ _ _ _ _ w630]
      frame "---------- Framework Operations ----------" {
        # "Dummy case to add a seperator in the Case Structure menu"
      }
      frame "", "Idle" {
        n194 = stacked-sequence {
          frame #0 {
            n195 = control-ref of="Enable Plating Cell"() -> (w358:refnum<vi>)
            n196 = shared-variable-read(refnum<k21> "ni.var.psp://z004551/CDL0100 ReadTags/Tnk6_Can_Plate" ("shared variable refnum in"), FALSE) -> (w368:bool)  [unwired: 1 in, 3 out]
            n197 = shared-variable-read(refnum<k21> "ni.var.psp://z004551/CDL0100 ReadWriteTags/HMI_Tank6_Enable" ("shared variable refnum in"), FALSE) -> (w355:bool)  [unwired: 1 in, 3 out]
            n198 = shared-variable-read(refnum<k21> "ni.var.psp://z004551/CDL0100 ReadWriteTags/HMI_Enable_BTnk3_Pump" ("shared variable refnum in"), FALSE) -> (w360:bool)  [unwired: 1 in, 3 out]
            n199 = shared-variable-read(refnum<k21> "ni.var.psp://z004551/CDL0100 ReadWriteTags/HMI_Tank5_Enable" ("shared variable refnum in"), FALSE) -> (w354:bool)  [unwired: 1 in, 3 out]
            n200 = Or(x=w355, y=w354) -> (x .or. y?=w353:bool)
            n201 = Or(x=w353, y=w360) -> (x .or. y?=w363:bool)
            n202 = case shown="False" w368 {
              tunnel: [T9."Disabled and Grayed Out" ("Disabled") T9."Enabled" ("Disabled")] -> w369
              frame False {
              }
              frame True {
              }
            }
            n203 = call "GrayOutButtonFromPSPVar.vi"("shared variable refnum in"=refnum<k21> "ni.var.psp://z004551/CDL0100 ReadWriteTags/HMI_Tank6_Drain", "Boolean in"=w358) -> ()  [unwired: 10 in]
            n204 = case shown="True" w363 {
              tunnel: [T9."Enabled" ("Disabled") T9."Disabled and Grayed Out" ("Disabled")] -> w362
              frame False {
              }
              frame True {
              }
            }
            n205 = control-ref of="Full Drain Plating Cell"() -> (w361:refnum<vi>)
            n206 = control-ref of="Start Cycle"() -> (w370:refnum<vi>)
            n207 = property class="Bool (strict)"(reference=w370, "DisabledEnum"=w369) -> ()  [unwired: 1 in, 2 out]
            n208 = property class="Bool (strict)"(reference=w361, "DisabledEnum"=w362) -> ()  [unwired: 1 in, 2 out]
          }
          frame #1 {
            n209 = shared-variable-read(refnum<k21> "ni.var.psp://z004551/CDL0100 ReadTags/IO_Bas_Tnk3_3Way_At_Recirc" ("shared variable refnum in"), FALSE) -> (w380:bool)  [unwired: 1 in, 3 out]
            n210 = shared-variable-read(refnum<k21> "ni.var.psp://z004551/CDL0100 ReadTags/IO_Bas_Tnk3_3Way_At_Open" ("shared variable refnum in"), FALSE) -> (w381:bool)  [unwired: 1 in, 3 out]
            n211 = shared-variable-read(refnum<k21> "ni.var.psp://z004551/CDL0100 ReadTags/IO_Bas_Tnk3_3Way_At_Closed" ("shared variable refnum in"), FALSE) -> (w384:bool)  [unwired: 1 in, 3 out]
            n212 = Or(x=w381, y=w380) -> (x .or. y?=w378:bool)
            "Sump Return" <- w378
            "Boolean 2" <- w378
            n213 = Or(x=w384, y=w381) -> (x .or. y?=w379:bool)
            "Return to sump" <- w379
            "Drain Tee Top" <- w379
            "Return to sump 2" <- w379
            "Process 1 Supply" <- w379
            n214 = Or(x=w379, y=w378) -> (x .or. y?=→"Boolean 5":bool)
          }
          frame #2 {
            n215 = shared-variable-read(refnum<k21> "ni.var.psp://z004551/CDL0100 ReadWriteTags/HMI_Tank6_Drain" ("shared variable refnum in"), FALSE) -> (w389:bool)  [unwired: 1 in, 3 out]
            n216 = shared-variable-read(refnum<k21> "ni.var.psp://z004551/CDL0100 ReadWriteTags/HMI_Enable_BTnk3_Pump" ("shared variable refnum in"), FALSE) -> (w390:bool)  [unwired: 1 in, 3 out]
            n217 = Or(x=w390, y=w389) -> (x .or. y?=→"SumpBottom":bool)
          }
          frame #3 {
            n218 = shared-variable-read(refnum<k21> "ni.var.psp://z004551/CDL0100 ReadTags/Rect11_12_CurrRecpStp" ("shared variable refnum in"), 0) -> (w396:i32)  [unwired: 1 in, 3 out]
            n219 = call-poly <userlib>:"Data Changed__ogtk.vi"("I32"=w396) -> ("Changed"=w397:bool)
            n220 = case shown="True" w397 {
              tunnel: w396 -> [_ w401]
              frame False {
              }
              frame True {
                w406 = 0.0 ("Scale.Range:Minimum")
                n221 = shared-variable-read(refnum<k21> "ni.var.psp://z004551/CDL0100 ReadWriteTags/HMI_Rect11_12_NumSteps" ("shared variable refnum in"), 0) -> (w400:i32)  [unwired: 1 in, 3 out]
                n222 = Less?(x=w401, y=w400) -> (x < y?=w413:bool)
                n223 = case shown="False" w413 {
                  tunnel: w401 -> [w418 w419]
                  tunnel: [w417 w419] -> w407
                  frame False {
                    n224 = Decrement(x=w418) -> (x-1=w417:i32)
                  }
                  frame True {
                  }
                }
                n225 = shared-variable-read(refnum<k21> "ni.var.psp://z004551/CDL0100 ReadWriteTags/HMI_Rct12_AMin_SetPnts" ("shared variable refnum in"), dbl[] []) -> (w408:dbl[])  [unwired: 1 in, 3 out]
                n226 = Index Array(array=w408, index=w407) -> (element=w404:dbl)
                n227 = shared-variable-read(refnum<k21> "ni.var.psp://z004551/CDL0100 ReadWriteTags/HMI_Rct11_AMin_SetPnts" ("shared variable refnum in"), dbl[] []) -> (w411:dbl[])  [unwired: 1 in, 3 out]
                n228 = Index Array(array=w411, index=w407) -> (element=w405:dbl)
                n229 = control-ref of="Right Anode Amp-min"() -> (w403:refnum<vi>)
                n230 = control-ref of="Left Anode Amp-min"() -> (w402:refnum<vi>)
                n231 = property class="Slide (strict)"(reference=w402, "Scale.Maximum"=w405, "Scale.Minimum"=w406) -> ()  [unwired: 1 in, 2 out]
                n232 = property class="Slide (strict)"(reference=w403, "Scale.Maximum"=w404, "Scale.Minimum"=w406) -> ()  [unwired: 1 in, 2 out]
              }
            }
          }
        }
        n233 = local read "Left Output On"() -> (w344:bool)
        n234 = local read "Right Output On"() -> (w345:bool)
        n235 = control-ref of="status"() -> (w351:refnum<vi>)
        n236 = Tick Count (ms)() -> (millisecond timer value=w346:u32)
        n237 = Subtract(x=w346, y=w347) -> (x-y=w349:u32)
        n238 = call <userlib>:"TAE Format Alarm Ticker.vi"("Alarm Ticker Ref"=w351) -> ()  [unwired: 15 in]
        n239 = Or(x=w344, y=w345) -> (x .or. y?=w343:bool)
        n240 = Greater?(x=w349, y=u32 500) -> (0:w342:bool)
        n241 = And(x=w343, y=w342) -> (x .and. y?=w341:bool)
        n242 = case shown="True" w341 {
          tunnel: w346 -> [_ w421]
          tunnel: [w420 w421] -> w348
          tunnel: w347 -> [w420 _]
          frame False {
          }
          frame True {
            n243 = shared-variable-read(refnum<k21> "ni.var.psp://z004551/CDL0100 ReadTags/Rect11_ActlVolts" ("shared variable refnum in"), 0.0) -> (w424:dbl)  [unwired: 1 in, 3 out]
            n244 = shared-variable-read(refnum<k21> "ni.var.psp://z004551/CDL0100 ReadTags/Rect12_ActlVolts" ("shared variable refnum in"), 0.0) -> (w423:dbl)  [unwired: 1 in, 3 out]
            n245 = Bundle(w424, w423) -> (→"Output Voltage":cluster{dbl, dbl})  [unwired: 1 in]
          }
        }
      }
      frame "Missing Message Handler", Default {
        # "Call this case if a message is received that is not handled \nby any other case. Typically this is a programming error\nas a result of a typo or unhandled message/missing message handler."
        n246 = Format Into String(format string="DevError: Missing message handler for '%s\" message." ("message"), w431) -> (resulting string=w429:string)  [unwired: 2 in, 1 out]
        n247 = One Button Dialog(message=w429) -> ()  [unwired: 2 out]
      }
      frame "Error" {
        # "General Error Case - this case is called if an error is passed using the error cluster below. Typically most new errors should be handed in each individual case and not passed in the rror cluster. If necessary a custom error handler case should be added and called from other cases."
        n248 = call <vilib>:"Simple Error Handler.vi"("error in (no error)"=w433) -> ()  [unwired: 1 in, 8 out]
      }
      frame "---------- Generic Operations ----------" {
        # "Dummy case to add a seperator in the Case Structure menu"
      }
      frame "Initialize" {
        n249 = stacked-sequence {
          seq-local: [_ w458 _ _ _ _] -> [_ _ w477 _ w521 w561]
          seq-local: [_ _ w475 _ _ _] -> [_ _ _ _ w516 w569]
          seq-local: [_ _ w474 _ _ _] -> [_ _ _ _ w514 w564]
          seq-local: [_ _ _ w505 _ _] -> [_ _ _ _ w515 _]
          seq-local: [_ _ _ w496 _ _] -> [_ _ _ _ w513 _]
          seq-local: [_ _ _ w495 _ _] -> [_ _ _ _ w512 _]
          seq-local: [_ _ _ w494 _ _] -> [_ _ _ _ w511 _]
          seq-local: [_ _ _ w493 _ _] -> [_ _ _ _ w510 _]
          frame #0 {
            n250 = shared-variable-read(refnum<k21> "ni.var.psp://z004551/CDL0100 ReadWriteTags/HMI_TNK6_SuckPmpFrac_Setpoint" ("shared variable refnum in"), 0.0) -> (w443:dbl)  [unwired: 1 in, 3 out]
            n251 = shared-variable-read(refnum<k21> "ni.var.psp://z004551/CDL0100 ReadWriteTags/HMI_Tnk6_Enable_SuckPump" ("shared variable refnum in"), FALSE) -> (w446:bool)  [unwired: 1 in, 3 out]
            n252 = shared-variable-read(refnum<k21> "ni.var.psp://z004551/CDL0100 ReadWriteTags/HMI_Tnk5_Rack_RPM" ("shared variable refnum in"), 0.0) -> (w457:dbl)  [unwired: 1 in, 3 out]
            n253 = shared-variable-read(refnum<k21> "ni.var.psp://z004551/CDL0100 ReadWriteTags/HMI_Tank6_Rack_Motor_Run" ("shared variable refnum in"), FALSE) -> (w456:bool)  [unwired: 1 in, 3 out]
            n254 = shared-variable-read(refnum<k21> "ni.var.psp://z004551/CDL0100 ReadWriteTags/HMI_Tank6_Motion_OverRide" ("shared variable refnum in"), FALSE) -> (w438:bool)  [unwired: 1 in, 3 out]
            n255 = shared-variable-read(refnum<k21> "ni.var.psp://z004551/CDL0100 ReadWriteTags/HMI_TNK6_Flow_Setpoint" ("shared variable refnum in"), 0.0) -> (w455:dbl)  [unwired: 1 in, 3 out]
            n256 = Multiply(x=w443, y=100.0) -> (x*y=w441:dbl)
            n257 = local write "Enable Suck Pump"(w446) -> ()
            n258 = local write "Rack RPM"(w457) -> ()
            n259 = local write "Enable Rack Motion"(w456) -> ()
            n260 = local write "Total Inflow (L/min)"(w455) -> ()
            n261 = local write "Suck Pump fraction of inflow"(w441) -> ()
            n262 = local write "Override Motion"(w438) -> ()
          }
          frame #1 {
            n263 = shared-variable-read(refnum<k21> "ni.var.psp://z004551/CDL0100 ReadWriteTags/HMI_Tank6_Drain" ("shared variable refnum in"), FALSE) -> (w461:bool)  [unwired: 1 in, 3 out]
            n264 = shared-variable-read(refnum<k21> "ni.var.psp://z004551/CDL0100 ReadWriteTags/HMI_Tnk5_Eductor_RPM" ("shared variable refnum in"), 0.0) -> (w469:dbl)  [unwired: 1 in, 3 out]
            n265 = shared-variable-read(refnum<k21> "ni.var.psp://z004551/CDL0100 ReadWriteTags/HMI_Tank6_Enable" ("shared variable refnum in"), FALSE) -> (w468:bool)  [unwired: 1 in, 3 out]
            n266 = local write "Full Drain Plating Cell"(w461) -> ()
            n267 = shared-variable-read(refnum<k21> "ni.var.psp://z004551/CDL0100 ReadWriteTags/HMI_Tank6_Eductor_Motors_Run" ("shared variable refnum in"), FALSE) -> (w472:bool)  [unwired: 1 in, 3 out]
            n268 = shared-variable-read(refnum<k21> "ni.var.psp://z004551/CDL0100 ReadWriteTags/HMI_Rect11_12_NumSteps" ("shared variable refnum in"), 0) -> (w458:i32)  [unwired: 1 in, 3 out]
            n269 = local write "Enable Plating Cell"(w468) -> ()
            n270 = local write "Eductor RPM"(w469) -> ()
            n271 = local write "Enable Eductor Motion"(w472) -> ()
          }
          frame #2 {
            w478 = 0.0
            n272 = shared-variable ".\\Local Variables.lvlib\\PT6_MO"() -> (w473:string)  [unwired: 1 in, 1 out]
            n273 = shared-variable-read(refnum<k21> "ni.var.psp://z004551/CDL0100 ReadWriteTags/HMI_Rct11_AMin_SetPnts" ("shared variable refnum in"), dbl[] []) -> (w475:dbl[])  [unwired: 1 in, 3 out]
            n274 = shared-variable-read(refnum<k21> "ni.var.psp://z004551/CDL0100 ReadWriteTags/HMI_Rct12_AMin_SetPnts" ("shared variable refnum in"), dbl[] []) -> (w474:dbl[])  [unwired: 1 in, 3 out]
            n275 = shared-variable-read(refnum<k21> "ni.var.psp://z004551/CDL0100 ReadWriteTags/HMI_BAS_TNK3_P_Setpoint" ("shared variable refnum in"), 0.0) -> (w484:dbl)  [unwired: 1 in, 3 out]
            n276 = for {
              N: w477 -> [_]
              tunnel: w474 -> [w489] mode=indexing
              shift-right: [w487] -> w476
              shift-left: w478 -> [w488]
              n277 = Add(x=w489, y=w488) -> (x+y=w487:dbl)
            }
            n278 = for {
              N: w477 -> [_]
              tunnel: w475 -> [w492] mode=indexing
              shift-right: [w490] -> w481
              shift-left: w478 -> [w491]
              n279 = Add(x=w492, y=w491) -> (x+y=w490:dbl)
            }
            n280 = local write "Supply Pressure (kPa)"(w484) -> ()
            n281 = local write "MO"(w473) -> ()
            n282 = local write "Total Amp*min L"(w481) -> ()
            n283 = local write "Total Amp*min R"(w476) -> ()
          }
          frame #3 {
            n284 = shared-variable-read(refnum<k21> "ni.var.psp://z004551/CDL0100 ReadWriteTags/HMI_Rct12_AFwd_SetPnts" ("shared variable refnum in"), dbl[] []) -> (w505:dbl[])  [unwired: 1 in, 3 out]
            n285 = shared-variable-read(refnum<k21> "ni.var.psp://z004551/CDL0100 ReadWriteTags/HMI_Rct11_FwdOffTm_SetPnts" ("shared variable refnum in"), dbl[] []) -> (w495:dbl[])  [unwired: 1 in, 3 out]
            n286 = shared-variable-read(refnum<k21> "ni.var.psp://z004551/CDL0100 ReadWriteTags/HMI_Rct11_FwdTm_SetPnts" ("shared variable refnum in"), dbl[] []) -> (w496:dbl[])  [unwired: 1 in, 3 out]
            n287 = shared-variable-read(refnum<k21> "ni.var.psp://z004551/CDL0100 ReadWriteTags/HMI_Rct11_BwdTm_SetPnts" ("shared variable refnum in"), dbl[] []) -> (w494:dbl[])  [unwired: 1 in, 3 out]
            n288 = shared-variable-read(refnum<k21> "ni.var.psp://z004551/CDL0100 ReadWriteTags/HMI_Rct11_BwdOffTm_SetPnts" ("shared variable refnum in"), dbl[] []) -> (w493:dbl[])  [unwired: 1 in, 3 out]
          }
          frame #4 {
            n289 = Subtract(x=10, y=w521) -> (x-y=w524:i32)
            n290 = Initialize Array(38, w521) -> (w523:i32[])
            n291 = Initialize Array(37, w524) -> (w522:i32[])
            n292 = Build Array (concatenate)(w523, w522) -> (w519:i32[])
            n293 = shared-variable-read(refnum<k21> "ni.var.psp://z004551/CDL0100 ReadWriteTags/HMI_Rct11_AFwd_SetPnts" ("shared variable refnum in"), dbl[] []) -> (w518:dbl[])  [unwired: 1 in, 3 out]
            n294 = for {
              N: 10 -> [_]
              tunnel: [w559] -> w509 mode=indexing
              tunnel: [w557] -> w508 mode=indexing
              tunnel: w518 -> [w555] mode=indexing
              tunnel: w516 -> [w552] mode=indexing
              tunnel: w515 -> [w549] mode=indexing
              tunnel: w514 -> [w546] mode=indexing
              tunnel: w513 -> [w543] mode=indexing
              tunnel: w512 -> [w540] mode=indexing
              tunnel: w511 -> [w537] mode=indexing
              tunnel: w510 -> [w534] mode=indexing
              i -> [w531]
              n295 = Number To Fractional String(number=w543, precision (6)=i16 1) -> (F-format string=w542:string)  [unwired: 2 in]
              n296 = Number To Fractional String(number=w546, precision (6)=i16 1) -> (F-format string=w545:string)  [unwired: 2 in]
              n297 = Number To Fractional String(number=w552, precision (6)=i16 1) -> (F-format string=w551:string)  [unwired: 2 in]
              n298 = Number To Fractional String(number=w549, precision (6)=i16 1) -> (F-format string=w548:string)  [unwired: 2 in]
              n299 = Number To Fractional String(number=w555, precision (6)=i16 1) -> (F-format string=w554:string)  [unwired: 2 in]
              n300 = Number To Fractional String(number=w540, precision (6)=i16 1) -> (F-format string=w539:string)  [unwired: 2 in]
              n301 = Number To Fractional String(number=w537, precision (6)=i16 1) -> (F-format string=w536:string)  [unwired: 2 in]
              n302 = Increment(x=w531) -> (x+1=w530:i32)
              n303 = Number To Decimal String(number=w531) -> (decimal integer string=w559:string)  [unwired: 1 in]
              n304 = Number To Fractional String(number=w534, precision (6)=i16 1) -> (F-format string=w533:string)  [unwired: 2 in]
              n305 = call "Build Text"("d"=w530) -> ("Result"=w532:string)  [unwired: 13 in, 1 out]
              n306 = Build Array("Active", w554, w551, w548, w545, w542, w539, w536, w533, w532) -> (w557:string[])
            }
            n307 = control-ref of="Rectifer Settings"() -> (w520:refnum<vi>)
            n308 = property class="MCListbox (strict)"(reference=w520, "ItemSyms"=w519, "RowHdrs[]"=w509, "ItemNames"=w508) -> ()  [unwired: 1 in, 2 out]
          }
          frame #5 {
            n309 = control-ref of="Rectifer Settings"() -> (w578:refnum<vi>)
            n310 = control-ref of="Right Anode Amp-min"() -> (w570:refnum<vi>)
            n311 = control-ref of="Left Anode Amp-min"() -> (w571:refnum<vi>)
            n312 = local read "Reverse Current Multiplier"() -> (w560:dbl)
            n313 = property class="MCListbox (strict)"(reference=w578) -> ("ItemNames"=w577:string[][])  [unwired: 1 in, 2 out]
            n314 = shared-variable-read(refnum<k21> "ni.var.psp://z004551/CDL0100 ReadTags/Rect11_12_CurrRecpStp" ("shared variable refnum in"), 0) -> (w562:i32)  [unwired: 1 in, 3 out]
            n315 = call "Calculate Plating Time.vi"("Num Steps"=w561, "ItemNames"=w577, "Reverse Current Multiplier"=w560) -> ("Right Anode Time"=w575:dbl, "Left Anode Time"=w576:dbl)  [unwired: 7 in]
            n316 = Less?(x=w562, y=w561) -> (x < y?=w572:bool)
            n317 = case shown="False" w572 {
              tunnel: w562 -> [w580 w581]
              tunnel: [w579 w581] -> w565
              frame False {
                n318 = Decrement(x=w580) -> (x-1=w579:i32)
              }
              frame True {
              }
            }
            n319 = local write "Right Time"(w575) -> ()
            n320 = local write "Left Time"(w576) -> ()
            n321 = Index Array(array=w569, index=w565) -> (element=w568:dbl)
            n322 = Index Array(array=w564, index=w565) -> (element=w563:dbl)
            n323 = property class="Slide (strict)"(reference=w571, "Scale.Maximum"=w568, "Scale.Minimum"=0.0 ("Scale.Range:Minimum")) -> ()  [unwired: 1 in, 2 out]
            n324 = property class="Slide (strict)"(reference=w570, "Scale.Maximum"=w563, "Scale.Minimum"=0.0 ("Scale.Range:Minimum")) -> ()  [unwired: 1 in, 2 out]
          }
        }
      }
      frame "Exit" {
        # "Destroy message queue >> this will halt the UI event handler loop"
        # "Stop the VI\n>> Perform any cleanup tasks in this message case.\n>> Clear display before closing."
        n325 = call <vilib>:"Destroy Message Queue.vi"("message queue in"=w583, "error in"=w584) -> ("error out"=w582:errorcluster)  [unwired: 11 in, 2 out]
        n326 = local write "status"("" ("Status")) -> ()
      }
      frame "---------- Application Operations ----------" {
        # "Dummy case to add a seperator in the Case Structure menu"
      }
      frame "Write_Tag" {
        n327 = call-poly <vilib>:"Write Message.vi"("error in"=w590, "data"=w588, "name"="WriteTag", "connection info in"=w591) -> ("error out"=w589:errorcluster)  [unwired: 6 in, 1 out]
      }
      frame "UpdateVPlotX" {
      }
      frame "DisplayLastHr" {
        n328 = call "Trace Variable 1 hour Popup.vi"("Tag"=w597) -> ()  [unwired: 11 in]
      }
      frame "UpdatePlatingMinutes" {
        n329 = local read "Reverse Current Multiplier"() -> (w598:dbl)
        n330 = Decimal String To Number(string=w600) -> (number=w599:i32)  [unwired: 2 in, 1 out]
        n331 = control-ref of="Rectifer Settings"() -> (w606:refnum<vi>)
        n332 = call "Assemble Rectifier Setting Changes for PLC.vi"("Num Steps"=w599, "Rect Number"=11, "error In"=w609, "Reverse Current Multiplier"=w598, "message queue in"=w605, "MulticolumnListbox in"=w606) -> ("Right Anode Mins"=w601:dbl, "Left Anode Mins"=w602:dbl, "Right AmpMin"=w603:dbl, "Left AmpMin"=w604:dbl, "error out"=w608:errorcluster)  [unwired: 1 in]
        n333 = local write "Total Amp*min L"(w604) -> ()
        n334 = local write "Total Amp*min R"(w603) -> ()
        n335 = local write "Left Time"(w602) -> ()
        n336 = local write "Right Time"(w601) -> ()
      }
      frame "Save_Recipe" {
        n337 = control-ref of="Rectifer Settings"() -> (w624:refnum<vi>)
        n338 = local read "Reverse Current Multiplier"() -> (w612:dbl)
        n339 = call "Convert RectifierListData to Arrays.vi"("MulticolumnListbox in"=w624, "error in (no error)"=w623) -> ("Left Amps"=w620:dbl[], "Right Amps"=w619:dbl[], "Left AmpMins"=w617:dbl[], "Right Amp Min"=w616:dbl[], "error out"=w615:errorcluster)  [unwired: 5 in, 4 out]
        n340 = shared-variable-read(refnum<k21> "ni.var.psp://z004551/CDL0100 ReadWriteTags/HMI_Rect11_12_NumSteps" ("shared variable refnum in"), 0) -> (w618:i32)  [unwired: 1 in, 3 out]
        n341 = call "Save Rectifier Recipe.vi"("Rev Mult"=w612, "Right AmpMins"=w616, "Left AmpMins"=w617, "error in"=w615, "Number Steps"=w618, "Right Amps"=w619, "Left Amps"=w620) -> ("error out"=w614:errorcluster, "name"=w610:string, "cancelled"=w611:bool)  [unwired: 2 in]
        n342 = case shown="True" w611 {
          tunnel: w610 -> [_ w625]
          frame False {
          }
          frame True {
            n343 = local write "Loaded Recipe"(w625) -> ()
          }
        }
      }
      frame "Load_A_Recipe" {
        n344 = call "BrowseRecipe.vi"() -> ("selected path"=w626:path)  [unwired: 9 in, 2 out]
        n345 = call "Read Rectifier Recipe.vi"("selected path"=w626, "error in"=w640) -> ("Left Amps"=w637:dbl[], "Left AmpMins"=w636:dbl[], "Canceled?"=w639:bool, "Num Steps"=w638:i32, "name"=w627:string, "Rev Mult"=w628:dbl, "Right Amps"=w635:dbl[], "Right AmpMins"=w633:dbl[], "error out"=w634:errorcluster)  [unwired: 5 in]
        n346 = case shown="False" w639 {
          tunnel: w638 -> [w647 _]
          tunnel: w637 -> [w661 _]
          tunnel: w636 -> [w660 _]
          tunnel: w635 -> [w659 _]
          tunnel: w634 -> [w658 w663]
          tunnel: w633 -> [w657 _]
          tunnel: [w643 w663] -> w632
          tunnel: w630 -> [w648 _]
          tunnel: w629 -> [w646 _]
          tunnel: w628 -> [w642 _]
          tunnel: w627 -> [w641 _]
          frame False {
            n347 = control-ref of="Rectifer Settings"() -> (w662:refnum<vi>)
            n348 = local write "Loaded Recipe"(w641) -> ()
            n349 = call "Write Pulse Rectifier Recipe to ListBox.vi"("Right AmpMins"=w657, "Left AmpMins"=w660, "Right Amps"=w659, "Left Amps"=w661, "error in (no error)"=w658, "Number Steps"=w647, "ListBox"=w662) -> ("error out"=w645:errorcluster)  [unwired: 4 in]
            n350 = local write "Reverse Current Multiplier"(w642) -> ()
            n351 = Number To Decimal String(number=w647) -> (decimal integer string=w649:string)  [unwired: 1 in]
            n352 = Bundle By Name(cluster=w648, "Data Type"=Data_Types."I32", "Name"="HMI_Rect11_12_NumSteps", "Value"=w649) -> (w653:T1)
            n353 = Flatten To String(anything=w653) -> (data string=w652:string)  [unwired: 3 in, 2 out]
            n354 = call <vilib>:"Send Local Message.vi"("message queue in"=w646, "message name"="Write_Tag", "message value"=w652, "error in"=w645) -> ("message queue out"=w651:T5, "error out"=w644:errorcluster)  [unwired: 9 in, 1 out]
            n355 = call <vilib>:"Send Local Message.vi"("message queue in"=w651, "message name"="UpdatePlatingMinutes", "message value"=w649, "error in"=w644) -> ("error out"=w643:errorcluster)  [unwired: 9 in, 2 out]
          }
          frame True {
          }
        }
      }
    }
  }
  n356 = call-poly <vilib>:"Get Connection Reference.vi"("error in"=w8, "connection info in"=w9) -> ("error out"=w12:errorcluster, "connection ID out"=w11:refnum<k5>)  [unwired: 8 out]
  n357 = TCP Close Connection(connection ID=w11, error in (no error)=w12) -> (error out=w14:errorcluster)  [unwired: 2 out]
  n358 = call <vilib>:"Error to Warning.vi"("1st Error to Convert"=w13, "error in"=w14) -> ("warning out"=w10:errorcluster)  [unwired: 3 in, 10 out]
  n359 = call <vilib>:"Simple Error Handler.vi"("error in (no error)"=w10) -> ()  [unwired: 4 in, 5 out]
